vi "assmbleVolume.vi"() -> ()   [LabVIEW 2010]
uses:
  scan_specification_cluster.ctl
  network_streaming_queues_cluster.ctl
panel:
  in  "network streaming queues":T1
  in  "error in (no error)":errorcluster
  in  "Queues":T2
  in  "assembler status":T3
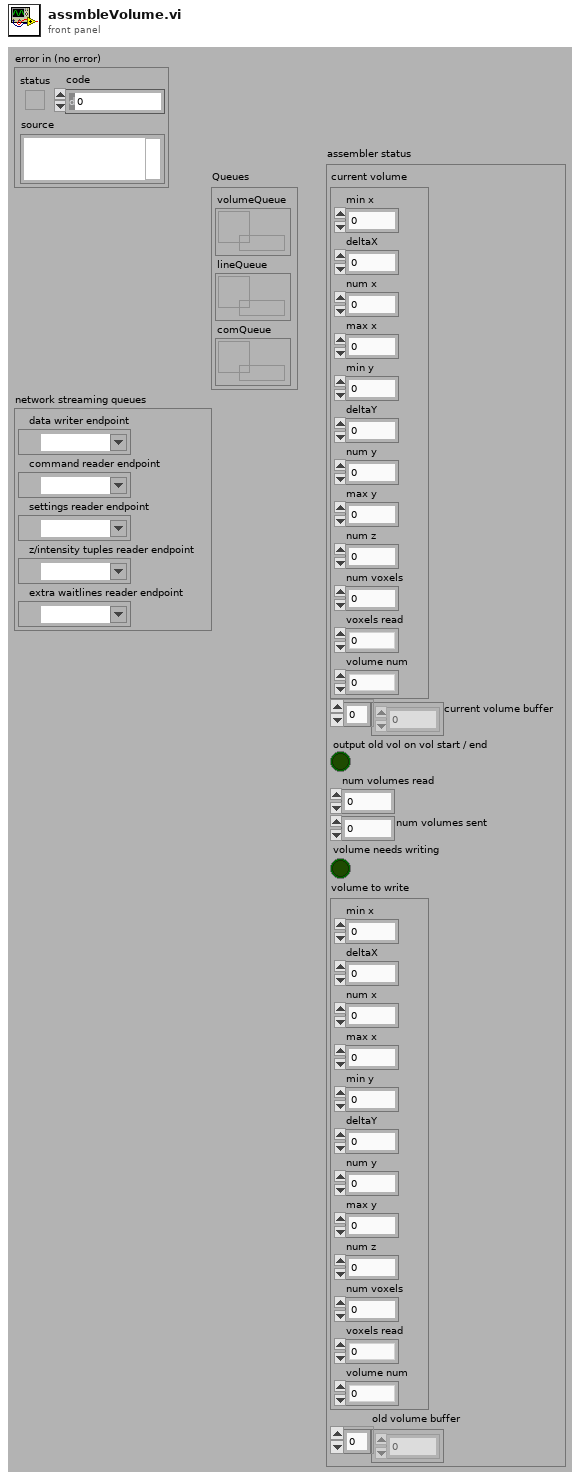
[diagram p1: front panel]
types:
  T1 = typedef "network_streaming_queues_cluster.ctl" = cluster{"data writer endpoint":refnum<k21>, "command reader endpoint":refnum<k21>, "settings reader endpoint":refnum<k21>, "z/intensity tuples reader endpoint":refnum<k21>, "extra waitlines reader endpoint":refnum<k21>}
  T2 = cluster{"volumeQueue":refnum<queue>, "lineQueue":refnum<queue>, "comQueue":refnum<queue>}
  T3 = cluster{"current volume":cluster{"min x":i16, "deltaX":dbl, "num x":u32, "max x":i16, "min y":i16, "deltaY":dbl, "num y":u32, "max y":i16, "num z":u32, "num voxels":u32, "voxels read":u32, "volume num":u32}, "current volume buffer":u32[], "output old vol on vol start / end":bool, "num volumes read":u32, "num volumes sent":u32, "volume needs writing":bool, "volume to write":cluster{"min x":i16, "deltaX":dbl, "num x":u32, "max x":i16, "min y":i16, "deltaY":dbl, "num y":u32, "max y":i16, "num z":u32, "num voxels":u32, "voxels read":u32, "volume num":u32}, "old volume buffer":u32[]}
  T4 = cluster{"start X":i16, "start Y":i16, "start Z":i16, "end X":i16, "end Y":i16, "end Z":i16, "num z":u8, "voxel data":u32[], "volume num":u32}[]
  T5 = cluster{"start X":i16, "start Y":i16, "start Z":i16, "end X":i16, "end Y":i16, "end Z":i16, "num z":u8, "voxel data":u32[], "volume num":u32}
  T6 = cluster{"min x":i16, "deltaX":dbl, "num x":u32, "max x":i16, "min y":i16, "deltaY":dbl, "num y":u32, "max y":i16, "num z":u32, "num voxels":u32, "voxels read":u32, "volume num":u32}
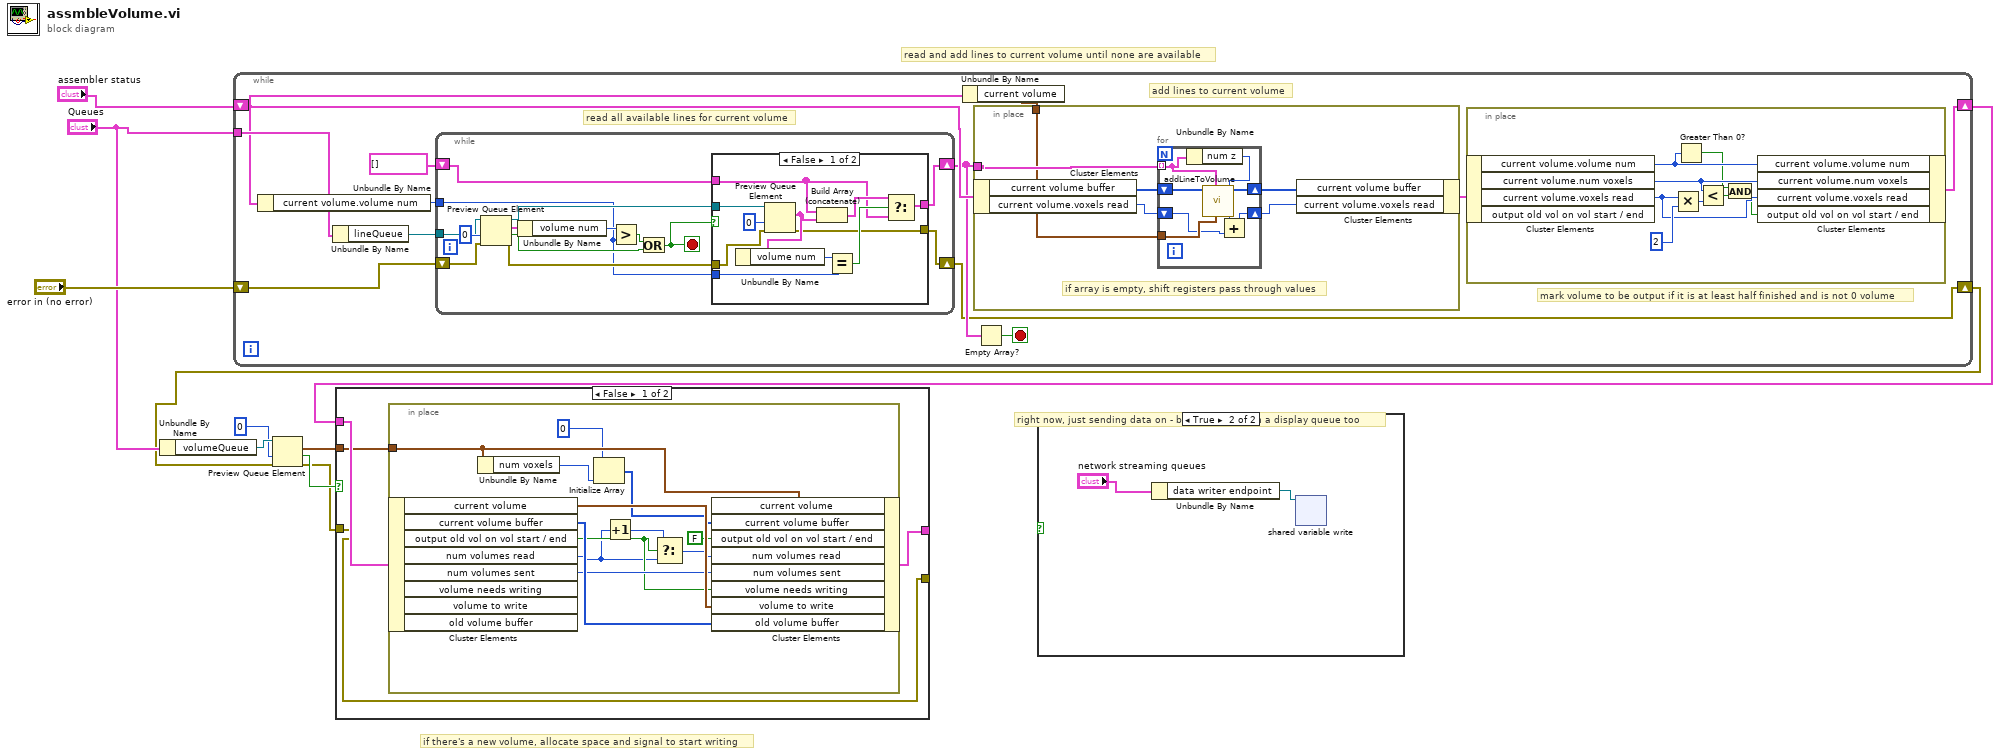
[diagram p0: block diagram]
diagram:
  # "right now, just sending data on - but could place in a display queue too"
  # "if there's a new volume, allocate space and signal to start writing"
  # "read and add lines to current volume until none are available"
  n1 = Unbundle By Name("Queues") -> ("volumeQueue"=w7:refnum<queue>)
  n2 = while {
    tunnel: "Queues" -> [w22]
    shift-right: [w15] -> w2
    shift-left: "assembler status" -> [w18]
    shift-right: [w12] -> w5
    shift-left: "error in (no error)" -> [w13]
    stop <- w11 stop-if-true
    # "mark volume to be output if it is at least half finished and is not 0 volume"
    # "add lines to current volume"
    # "read all available lines for current volume"
    n3 = Unbundle By Name(w18) -> ("current volume.volume num"=w20:u32)
    n4 = Unbundle By Name(w22) -> ("lineQueue"=w21:refnum<queue>)
    n5 = while {
      tunnel: w21 -> [w50]
      tunnel: w20 -> [w45]
      shift-right: [w47] -> w14
      shift-left: T4 [] -> [w46]
      shift-right: [w44] -> w12
      shift-left: w13 -> [w56]
      stop <- w51 stop-if-true
      n6 = Preview Queue Element(queue=w50, timeout in ms (-1)=0, error in (no error)=w56) -> (queue out=w48:refnum<queue>, element=w55:T5, timed out?=w52:bool, error out=w49:errorcluster)
      n7 = Unbundle By Name(w55) -> ("volume num"=w54:u32)
      n8 = Greater?(x=w54, y=w45) -> (0:w53:bool)
      n9 = Or(x=w53, y=w52) -> (x .or. y?=w51:bool)
      n10 = case shown="False" w51 {
        tunnel: w48 -> [w68 _]
        tunnel: w49 -> [w67 w69]
        tunnel: [w59 w70] -> w47
        tunnel: w46 -> [w60 w70]
        tunnel: w45 -> [w63 _]
        tunnel: [w58 w69] -> w44
        frame False {
          n11 = Preview Queue Element(queue=w68, timeout in ms (-1)=0, error in (no error)=w67) -> (element=w65:T5, error out=w58:errorcluster)  [unwired: 2 out]
          n12 = Unbundle By Name(w65) -> ("volume num"=w64:u32)
          n13 = Build Array (concatenate)(w60, w65) -> (w61:T4)
          n14 = Equal?(x=w64, y=w63) -> (x = y?=w62:bool)
          n15 = Select(t=w61, s=w62, f=w60) -> (s? t:f=w59:T4)
        }
        frame True {
        }
      }
    }
    n16 = Unbundle By Name(w18) -> ("current volume"=w17:T6)
    n17 = in-place {
      in-place-border: w14 -> [w36]
      in-place-border: w17 -> [w33]
      # "if array is empty, shift registers pass through values"
      n18 = in-place-cluster #1(w18) -> ("current volume buffer"=w35:u32[], "current volume.voxels read"=w32:u32)
      n19 = for {
        tunnel: w36 -> [w40] mode=indexing
        tunnel: w33 -> [w43]
        shift-right: [w41] -> w34
        shift-left: w35 -> [w42]
        shift-right: [w37] -> w31
        shift-left: w32 -> [w38]
        n20 = Unbundle By Name(w40) -> ("num z"=w39:u8)
        n21 = call "addLineToVolume.vi"("current volume"=w43, "line"=w40, "volume buffer"=w42) -> ("volume buffer out"=w41:u32[])  [unwired: 6 in, 2 out]
        n22 = Add(x=w39, y=w38) -> (x+y=w37:u32)
      }
      n23 = in-place-cluster #1("current volume buffer"=w34, "current volume.voxels read"=w31) -> (w16:T3)
    }
    n24 = Empty Array?(array=w14) -> (empty?=w11:bool)
    n25 = in-place {
      n26 = in-place-cluster #2(w16) -> ("current volume.volume num"=w24:u32, "current volume.num voxels"=w27:u32, "current volume.voxels read"=w26:u32)  [unwired: 1 out]
      n27 = Multiply(x=w26, y=u32 2) -> (x*y=w29:u32)
      n28 = Greater Than 0?(x=w24) -> (x > 0?=w23:bool)
      n29 = Less?(x=w27, y=w29) -> (x < y?=w28:bool)
      n30 = And(x=w23, y=w28) -> (x .and. y?=w25:bool)
      n31 = in-place-cluster #2("current volume.volume num"=w24, "current volume.num voxels"=w27, "current volume.voxels read"=w26, "output old vol on vol start / end"=w25) -> (w15:T3)
    }
  }
  n32 = Preview Queue Element(queue=w7, timeout in ms (-1)=0, error in (no error)=w5) -> (element=w1:T6, timed out?=w4:bool, error out=w3:errorcluster)  [unwired: 1 out]
  n33 = case shown="False" w4 {
    tunnel: w3 -> [w71 w87]
    tunnel: w2 -> [w74 w88]
    tunnel: w1 -> [w73 _]
    tunnel: [w72 w88] -> _
    tunnel: [w71 w87] -> _
    frame False {
      n34 = in-place {
        in-place-border: w73 -> [w79]
        n35 = in-place-cluster #3(w74) -> ("current volume"=w85:T6, "current volume buffer"=w86:u32[], "output old vol on vol start / end"=w83:bool, "num volumes read"=w80:u32, "num volumes sent"=w84:u32)  [unwired: 3 out]
        n36 = Unbundle By Name(w79) -> ("num voxels"=w78:u32)
        n37 = Initialize Array(u32 0, w78) -> (w76:u32[])
        n38 = Increment(x=w80) -> (x+1=w81:u32)
        n39 = Select(t=w81, s=w83, f=w80) -> (s? t:f=w82:u32)
        n40 = in-place-cluster #3("current volume"=w79, "current volume buffer"=w76, "output old vol on vol start / end"=FALSE, "num volumes read"=w82, "num volumes sent"=w84, "volume needs writing"=w83, "volume to write"=w85, "old volume buffer"=w86) -> (w72:T3)
      }
    }
    frame True {
    }
  }
  n41 = case shown="True" {
    selector: _ -> [_ _]
    frame False {
    }
    frame True {
      n42 = Unbundle By Name("network streaming queues") -> ("data writer endpoint"=w89:refnum<k21>)
      n43 = shared-variable-write(w89) -> ()  [unwired: 3 in, 3 out]
    }
  }
